vi "write shared data.vi"(8 "error in (no error)":errorcluster, 10 "shared data":T1, 11 "Item Ref in":T2 format="%.0x") -> (0 "error out":errorcluster, 3 "Item Ref out":T2 format="%.0x")   [LabVIEW 2017, in "DSF System Explorer.lvlib"]
uses:
  DSF System Explorer.lvlib
  <vilib>/NI Veristand/Custom Device API/Custom Device Item Ref.ctl
  shared data.ctl
  DSF Core.lvlibp/Classes/Configuration/Configuration Session.lvclass
  <vilib>/NI Veristand/Custom Device API/Custom Device API.lvlib
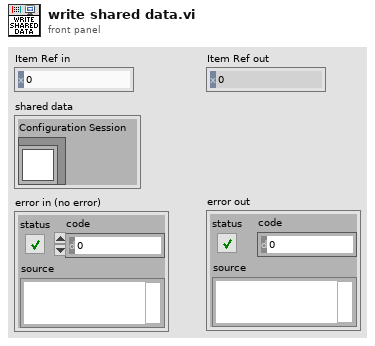
[diagram p1: front panel]
types:
  T1 = typedef "DSF System Explorer.lvlib/shared data.ctl" = cluster{"Configuration Session":refnum<class "Configuration Session.lvclass">}
  T2 = typedef "Custom Device API.lvlib/Custom Device Item Ref.ctl" = u64
  T3 = typedef "DSF System Explorer.lvlib/shared data ref.ctl" = refnum<data-value>
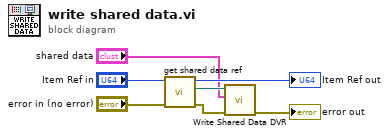
[diagram p0: block diagram]
diagram:
  n1 = call "get shared data ref.vi"("error in (no error)"="error in (no error)", "Node Ptr"="Item Ref in") -> ("error out"=w4:errorcluster, "shared data ref"=w3:T3, "Item Ref out"=→"Item Ref out":T2)  [unwired: 7 in]
  n2 = call "Write Shared Data DVR.vi"("error in (no error)"=w4, "shared data"="shared data", "Shared Data DVR in"=w3) -> ("error out"=→"error out":errorcluster)  [unwired: 7 in, 1 out]
